vi "曲线采集.vi"(0 "曲线引用":refnum<vi>, 5 "曲线索引":i32, 7 "X":sgl, 9 "Y":sgl, 11 "错误输入（无错误）":errorcluster) -> (4 "曲线引用Out":refnum<vi>, 15 "错误输出":errorcluster)   [LabVIEW 2018]
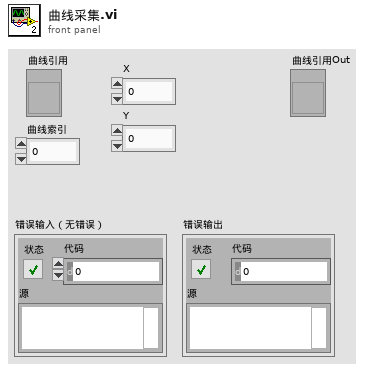
[diagram p1: front panel]
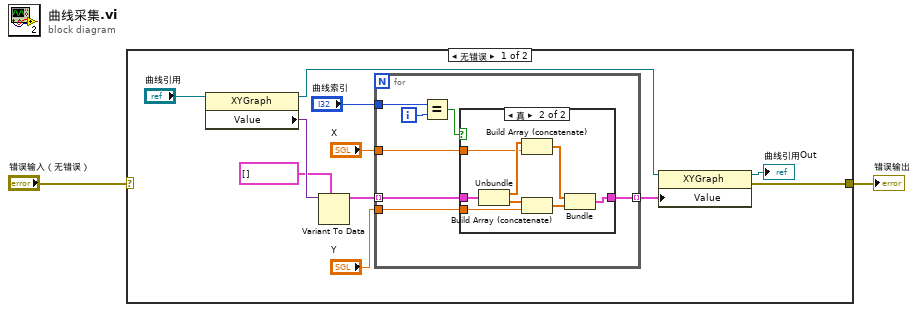
[diagram p0: block diagram]
diagram:
  n1 = case shown="无错误" "错误输入（无错误）" {
    selector: "错误输入（无错误）" -> [_ w30]
    tunnel: [w7 w30] -> w2
    frame No Error {
      n2 = property class="XYGraph"(reference="曲线引用") -> (reference out=w4:refnum<vi>, "Value"=w13:variant)  [unwired: 1 in, 1 out]
      n3 = Variant To Data(type=cluster{"X":dbl[], "Y":dbl[]}[] [], Variant=w13) -> (data=w11:cluster{"X":dbl[], "Y":dbl[]}[])  [unwired: 1 in, 1 out]
      n4 = for {
        tunnel: w11 -> [w17] mode=indexing
        tunnel: "曲线索引" -> [w19]
        tunnel: [w16] -> w8 mode=indexing
        tunnel: "X" -> [w15]
        tunnel: "Y" -> [w14]
        i -> [w20]
        n5 = Equal?(x=w19, y=w20) -> (x = y?=w18:bool)
        n6 = case shown="真" w18 {
          tunnel: w17 -> [w21 w29]
          tunnel: [w21 w22] -> w16
          tunnel: w15 -> [_ w27]
          tunnel: w14 -> [_ w25]
          frame False {
          }
          frame True {
            n7 = Unbundle(w29) -> ("X"=w28:dbl[], "Y"=w26:dbl[])
            n8 = Build Array (concatenate)(w28, w27) -> (w24:dbl[])
            n9 = Build Array (concatenate)(w26, w25) -> (w23:dbl[])
            n10 = Bundle(w24, w23) -> (w22:cluster{dbl[], dbl[]})  [unwired: 1 in]
          }
        }
      }
      n11 = property class="XYGraph"(reference=w4, "Value"=w8) -> (reference out=→"曲线引用Out":refnum<vi>, error out=w7:errorcluster)  [unwired: 1 in]
    }
    frame Error {
    }
  }
  "错误输出" <- w2
